vi "Is COMxx port present.vi"(8 "error in (no error)":errorcluster, 11 "Comport":string) -> (0 "error out":errorcluster, 3 "Comport found":bool)   [LabVIEW 2013]
panel:
  out "standard output":string="USB\\VID_1D6B&PID_0104&MI_02\\7&10A9E9AA&0&0002               : Gadget Serial (COM8)\r\n1 matching device(s) found.\r\n"
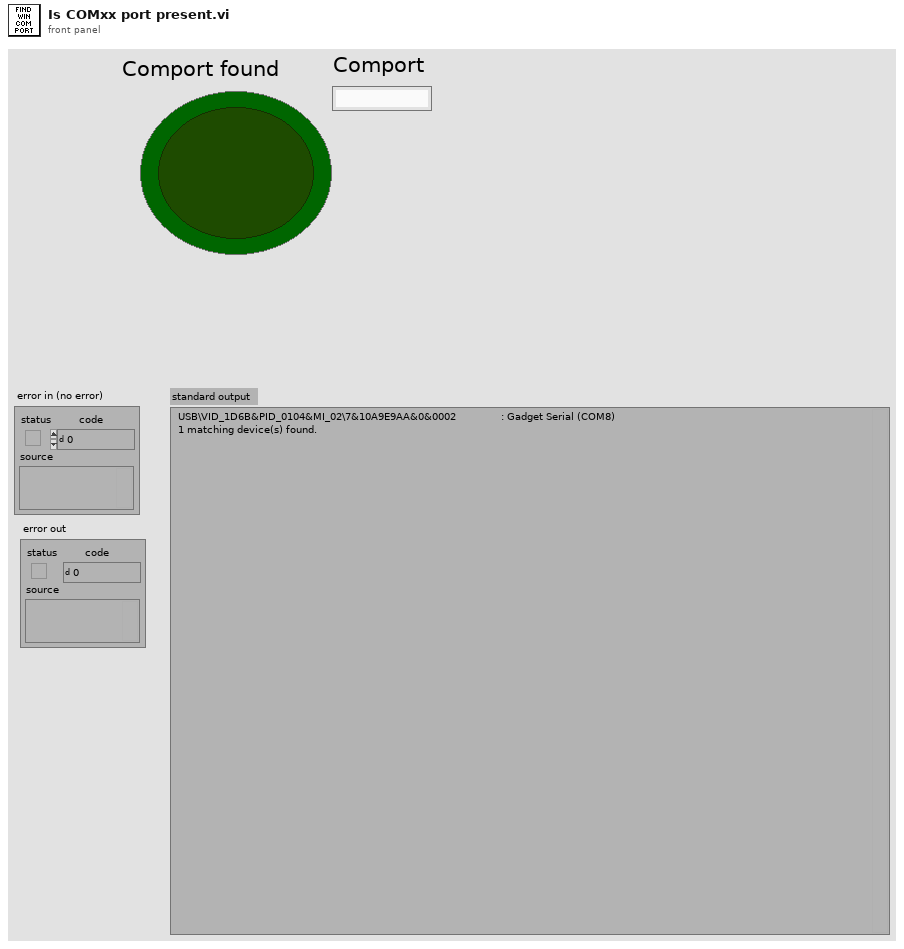
[diagram p1: front panel]
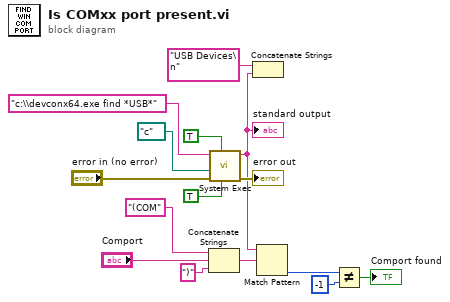
[diagram p0: block diagram]
diagram:
  n1 = Concatenate Strings("(COM" ("string"), "Comport", ")" ("string")) -> (w4:string)
  n2 = call <vilib>:"System Exec.vi"("run minimized? (F)"=TRUE, "wait until completion? (T)"=TRUE, "error in (no error)"="error in (no error)", "working directory"=path "c:/", "command line"="c:\\devconx64.exe find *USB*") -> ("error out"=→"error out":errorcluster, "standard output"=w2:string)  [unwired: 3 in, 2 out]
  "standard output" <- w2
  n3 = Concatenate Strings("USB Devices\n" ("string"), w2) -> ()  [unwired: 1 out]
  n4 = Match Pattern(string=w2, regular expression=w4) -> (offset past match=w10:i32)  [unwired: 1 in, 3 out]
  n5 = Not Equal?(x=w10, y=-1) -> (x != y?=→"Comport found":bool)
